vi "Str_Data - Mod.vi"(3 "Err str":string, 4 "Msg":T1 {"ID" format="%x"; "MSGTYPE" items=["STATUS"=128, "EXTENDED"=2, "RTR"=1, "DATA MSG"=0]; "aDATA" format="%x"}, 6 "string":string) -> (1 "str out":string)   [LabVIEW 2017]
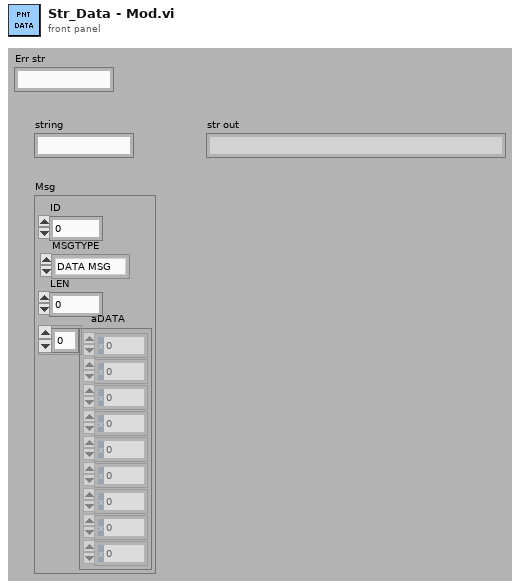
[diagram p1: front panel]
types:
  T1 = cluster{"ID":u32, "MSGTYPE":u8, "LEN":u8, "aDATA":u8[]}
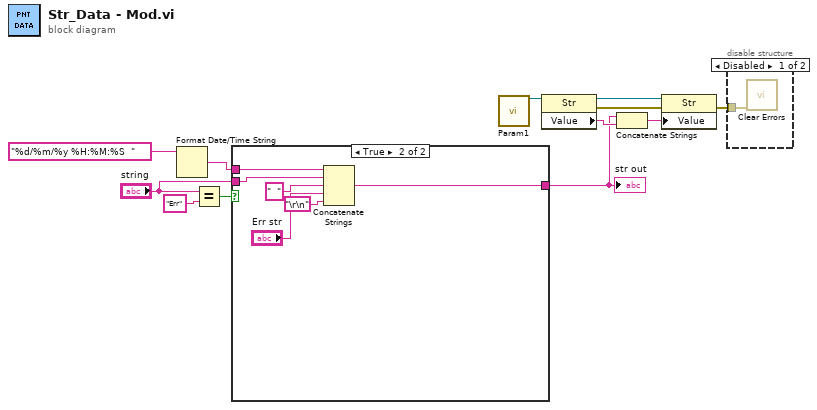
[diagram p0: block diagram]
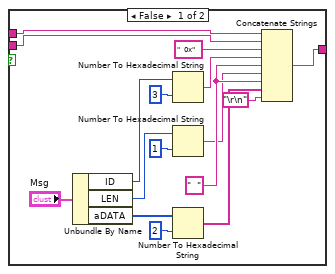
[diagram p3: hidden frame]
diagram:
  n1 = Format Date/Time String(time format string (%c)="%d/%m/%y %H:%M:%S  ") -> (date/time string=w12:string)  [unwired: 2 in]
  n2 = Equal?(x="string", y="Err") -> (x = y?=w8:bool)
  n3 = case shown="True" w8 {
    tunnel: w12 -> [w21 w33]
    tunnel: [w15 w34] -> w2
    tunnel: "string" -> [w14 w32]
    frame False {
      w25 = "  " ("string")
      n4 = Unbundle By Name("Msg") -> ("ID"=w17:u32, "LEN"=w18:u8, "aDATA"=w26:u8[])
      n5 = Number To Hexadecimal String(1:i16 3 ("width (-)"), 2:w17) -> (0:w23:string)
      n6 = Number To Hexadecimal String(1:i16 1 ("width (-)"), 2:w18) -> (0:w24:string)
      n7 = Number To Hexadecimal String(1:i16 2 ("width (-)"), 2:w26) -> (0:w27:string[])
      n8 = Concatenate Strings(w21, w14, "  0x" ("string"), w23, w25, w24, w25, w27, "\r\n") -> (w15:string)
    }
    frame True {
      n9 = Concatenate Strings(w33, w32, "  " ("string"), "Err str", "\r\n") -> (w34:string)
    }
  }
  "str out" <- w2
  n10 = call "Param1.vi"() -> ("str out"=w3:refnum<vi>)  [unwired: 18 in, 1 out]
  n11 = property class="Str"(reference=w3) -> (reference out=w6:refnum<vi>, error out=w5:errorcluster, "Value"=w7:string)  [unwired: 1 in]
  n12 = Concatenate Strings(w2, w7) -> (w4:string)
  n13 = property class="Str"(reference=w6, error in=w5, "Value"=w4) -> (error out=w1:errorcluster)  [unwired: 1 out]
  n14 = disable-structure shown="Disabled" {
    disable-tunnel: w1 -> [w35 _]
    frame Disabled {
      n15 = call <vilib>:"Clear Errors.vi"("error in (no error)"=w35) -> ()  [unwired: 5 in, 2 out]
    }
    frame Enabled {
    }
  }
